vi "Assignment_01_1.vi"() -> ()   [LabVIEW 2023]
panel:
  out "Digital_Code":dbl
  in  "Resolution(bits)":dbl=8.0
  in  "Voltage_Range(V)":dbl=10.0
  in  "Analog_Data(V)":dbl
  # "Analog To Digital Converter"
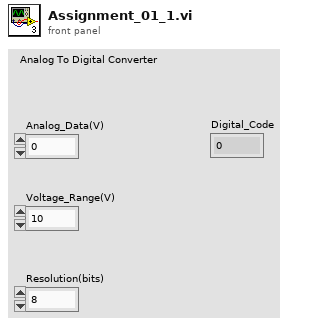
[diagram p1: front panel]
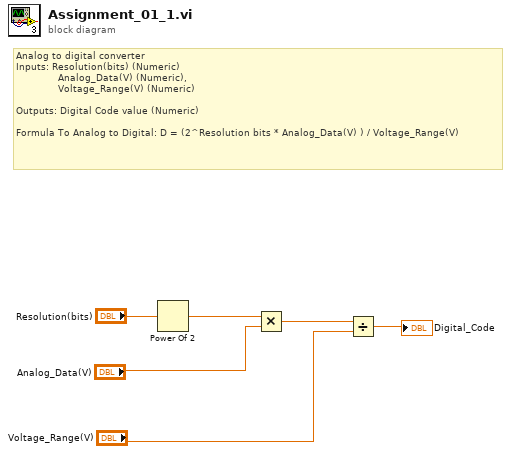
[diagram p0: block diagram]
diagram:
  # "Analog to digital converter\nInputs: Resolution(bits) (Numeric)\n              Analog_Data(V) (Numeric),\n              Voltage_Range(V) (Numeric)\n\nOutputs: Digital Code value (Numeric)\n\nFormula To Analog to Digital: D = (2^Resolution bits * Analog_Data(V) ) / Voltage_Range(V)"
  n1 = Power Of 2(x="Resolution(bits)") -> (2^x=w5:dbl)
  n2 = Multiply(x=w5, y="Analog_Data(V)") -> (x*y=w3:dbl)
  n3 = Divide(x=w3, y="Voltage_Range(V)") -> (x/y=→"Digital_Code":dbl)
